vi "TEST_I2C_ADS1115_ESP8266.vi"() -> ()   [LabVIEW 2014]
uses:
  <vilib>/MakerHub/LINX/Private/Device/Type Defs/TCP Config.ctl
  User Defined/I2C_Platform_Selector.ctl
  <vilib>/MakerHub/LINX/Public/Utilities/Open TCP.vi
  <vilib>/MakerHub/LINX/LMH-LINX.lvlib
  <vilib>/MakerHub/LINX/Private/Device/Device.lvlib
panel:
  out "mV_out":u16
  out "(hi.lo)":i16 format="%.0b"
  out "mV out":dbl format="%#_f"
  in  "stop":bool
  out "Waveform Chart":dbl[](graph)
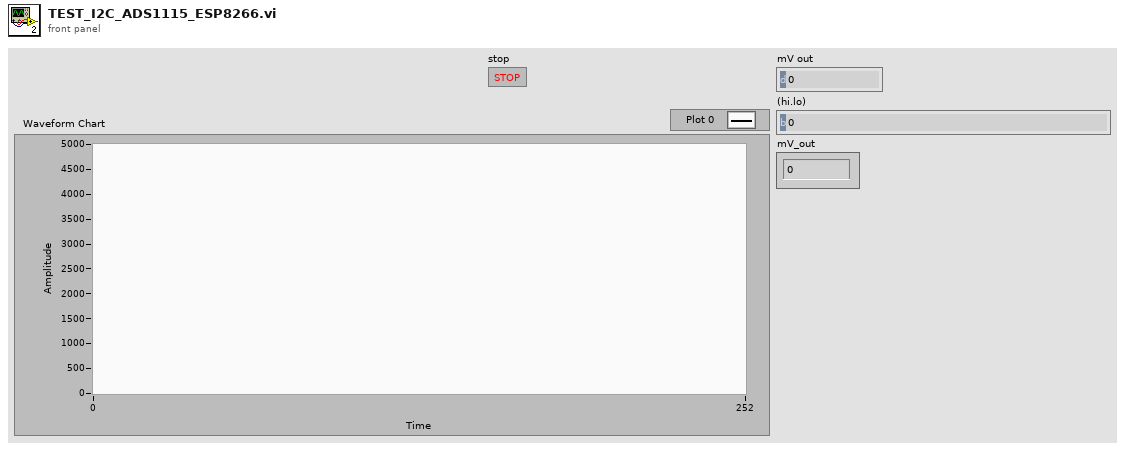
[diagram p1: front panel]
types:
  T1 = typedef "I2C_Platform_Selector.ctl" = enum16{"ESP8266-I2C", "Raspberry Pi-I2C"}
  T2 = typedef "LMH-LINX.lvlib/Device.lvlib/TCP Config.ctl" = cluster{"IP Address":string, "Port":u16}
  T3 = cluster{"ADS1015-Channel Selector":enum8{"DIFF-AI0-AI1", "DIFF-AI0-AI3", "DIFF-AI1-AI3", "DIFF-AI2-AI3", "Single Ended - AI0", "Single Ended - AI1", "Single Ended - AI2", "Single Ended - AI3"}, "ADS1015 -Gain & Scale":enum8{"FS=+/-6.144 V", "FS=+/-4.096 V", "FS=+/-2.048 V", "FS=+/-1.024 V", "FS=+/-0.512 V", "FS=+/-0.256-A V", "FS=+/-0.256-B V", "FS=+/-0.256-C V"}, "ADS1015- Acquire Mode":enum16{"Continuous Conversion Mode", "Single Shot Mode"}, "ADS1015 Sample Rate":enum8{"128 SPS", "250 SPS", "490 SPS", "920 SPS", "1600 SPS", "2400 SPS", "3300 SPS", "3300 SPS A"}}
  T4 = typedef "LMH-LINX.lvlib/LINX Ref.ctl" = cluster{"IO":T5, "Interface":T6, "LINX Device Config":T7}
  T5 = typedef "LMH-LINX.lvlib/Platform.ctl" = enum16{"Remote", "Local"}
  T6 = typedef "LMH-LINX.lvlib/Interface.ctl" = enum16{"Serial", "TCP"}
  T7 = typedef "LMH-LINX.lvlib/Device.lvlib/LINX Device Config.ctl" = cluster{"Interface":T6, "COM Port":refnum<visa-resource-name>, "TCP Configuration":T2, "Device Family":u8, "Device ID":u8, "Device Name":string, "TCP Ref":refnum<k5>, "Channels":T8}
  T8 = typedef "LMH-LINX.lvlib/Channels.ctl" = cluster{"DI":u8[], "DO":u8[], "AI":u8[], "AO":u8[], "PWM":u8[], "QE":u8[], "UART":u8[], "I2C 2":u8[], "SPI":u8[], "CAN":u8[], "Servo":u8[], "AI Ref (V)":dbl, "AI Resolution (Bits)":u8, "AO Ref (V)":dbl, "AO Resolution (Bits)":u8}
  T9 = enum8{"FS=+/-6.144 V", "FS=+/-4.096 V", "FS=+/-2.048 V", "FS=+/-1.024 V", "FS=+/-0.512 V", "FS=+/-0.256-A V", "FS=+/-0.256-B V", "FS=+/-0.256-C V"}
  T10 = enum8{"DIFF-AI0-AI1", "DIFF-AI0-AI3", "DIFF-AI1-AI3", "DIFF-AI2-AI3", "Single Ended - AI0", "Single Ended - AI1", "Single Ended - AI2", "Single Ended - AI3"}
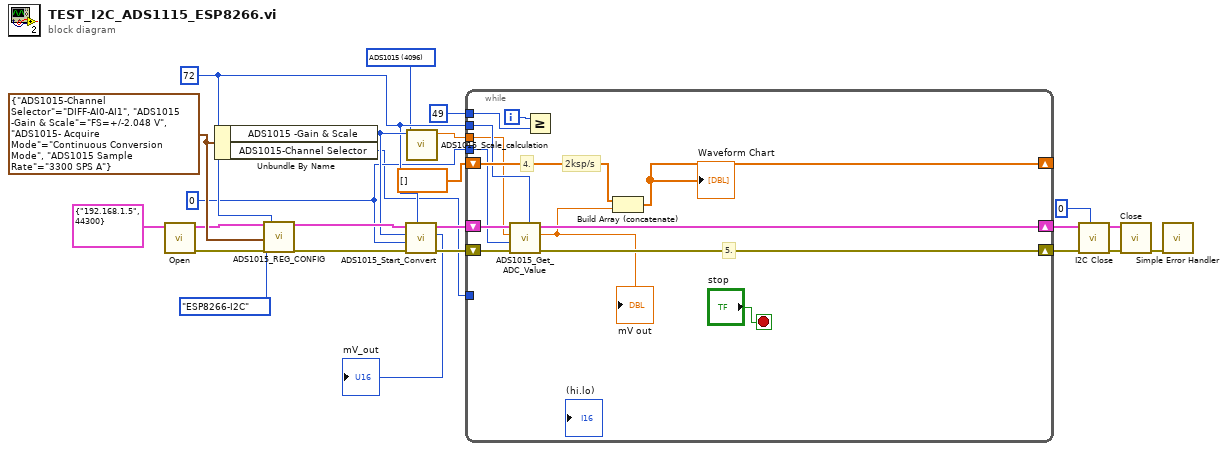
[diagram p0: block diagram]
diagram:
  w2 = 4096 items=["ADS1015"=4096, "AD1115"=65536] ("IC Selector")
  w5 = u8 0 ("I2C Channel (RPI)")
  w7 = u8 72 ("I2C Slave Address (0)")
  w17 = T3 {"ADS1015-Channel Selector"=enum."DIFF-AI0-AI1", "ADS1015 -Gain & Scale"=enum."FS=+/-2.048 V", "ADS1015- Acquire Mode"=enum."Continuous Conversion Mode", "ADS1015 Sample Rate"=enum."3300 SPS A"} ("ADS1015 Reg Config")
  n1 = call-poly <vilib>:"Open.vi"("TCP Configuration"=T2 {"IP Address"="192.168.1.5", "Port"=44300}) -> ("Error Out"=w8:errorcluster, "LINX Resource"=w9:T4)  [unwired: 8 in, 1 out]
  n2 = Unbundle By Name(w17) -> ("ADS1015 -Gain & Scale"=w16:T9, "ADS1015-Channel Selector"=w1:T10)
  n3 = call "ADS1015_REG_CONFIG.vi"("LINX Resource in"=w9, "ADS1015 Reg Config"=w17, "I2C_Channel_platform"=I2C_Platform_Selector."ESP8266-I2C", "Error In"=w8, "I2C Slave Address (0)"=w7) -> ("LINX Resource out"=w20:T4, "Error Out"=w23:errorcluster)  [unwired: 13 in]
  n4 = call "ADS1015_Start_Convert.vi"("I2C Slave Address (0)"=w7, "error in (no error)"=w23, "I2C_Channel_platform"=w5, "Scale mV"=w16, "LINX Resource in"=w20) -> ("error out"=w22:errorcluster, "mV_out"=→"mV_out":u16, "LINX Resource out"=w19:T4)  [unwired: 4 in]
  n5 = call "ADS1015_Scale_calculation.vi"("IC Selector"=w2, "ADS1015 -Gain & Scale"=w16) -> ("Scale Value (mV)"=w18:dbl)  [unwired: 9 in]
  n6 = while {
    shift-right: [w32] -> w14
    shift-left: w19 -> [w33]
    shift-right: [w37] -> w12
    shift-left: w22 -> [w36]
    shift-right: [w28] -> _
    shift-left: dbl[] [] -> [w35]
    tunnel: w7 -> [w31]
    tunnel: w18 -> [w25]
    tunnel: 49 ("y") -> [w29]
    tunnel: w5 -> [w26]
    tunnel: w1 -> [_]
    i -> [w34]
    stop <- "stop" stop-if-true
    # "2ksp/s"
    # "5."
    # "4."
    n7 = call "ADS1015_Get_ADC_Value.vi"("I2C Slave Address (0)"=w31, "error in (no error)"=w36, "I2C_Channel_platform"=w26, "Scale Value (mV)"=w25, "LINX Resource in"=w33) -> ("error out"=w37:errorcluster, "mV out"=w30:dbl, "LINX Resource"=w32:T4)  [unwired: 3 in, 1 out]
    "mV out" <- w30
    n8 = Greater Or Equal?(x=w34, y=w29) -> ()  [unwired: 1 out]
    n9 = Build Array (concatenate)(w35, w30) -> (w28:dbl[])
    "Waveform Chart" <- w28
  }
  n10 = call <vilib>:"I2C Close.vi"("I2C Channel (0)"=u8 0, "Error In"=w12, "LINX Resource"=w14) -> ("Error Out"=w11:errorcluster, "LINX Resource"=w13:T4)  [unwired: 7 in]
  n11 = call <vilib>:"Close.vi"("Error In"=w11, "LINX Resource"=w13) -> ("Error Out"=w24:errorcluster)  [unwired: 9 in]
  n12 = call <vilib>:"Simple Error Handler.vi"("error in (no error)"=w24) -> ()  [unwired: 4 in, 5 out]
